vi "maincapactor1.vi"() -> ()   [LabVIEW 2024]
panel:
  out "dup directory path":path
  in  "GPIB address magnet":string
  in  "GPIB address Temp Controler":string
  in  "GPIB address CapBridge":string
  in  "Wait (minute)":u32
  in  "No of Temp Steps":i16
  in  "folder name to save files":string
  out "outputtemp":dbl[](array[numeric]) format="%.2f"
  out "outputdc":dbl[](array[numeric]) format="%.2f"
  out "outputcapacitor":dbl[](array[numeric]) format="%.2f"
  out "field":dbl[](array[numeric]) format="%.2f"
  out "Current Temp":dbl format="%.3f"
  in  "Increasing \nTemp step":bool=TRUE
  in  "Temperature\nInterval":dbl format="%.3f"
  in  "Initial Temp C":dbl format="%.3f"
  # "Help:\n1. write the folder name to save the files.The file name will \nbe the temperature in the given folder.\n2.Write the GPIB address of all the instruments before running\nthe program.\n3. Give the initial temperature and the temperature interval \nand the total number of steps.\n4.Check whether you want to increase the temperature or\ndecrease.\n5.Write the time to be waited to let the tempetature controller\nequilibrate.\n6.Once the speps 1 through 5 is done run the experiment."
  # "Decreasing\nTemp Step"
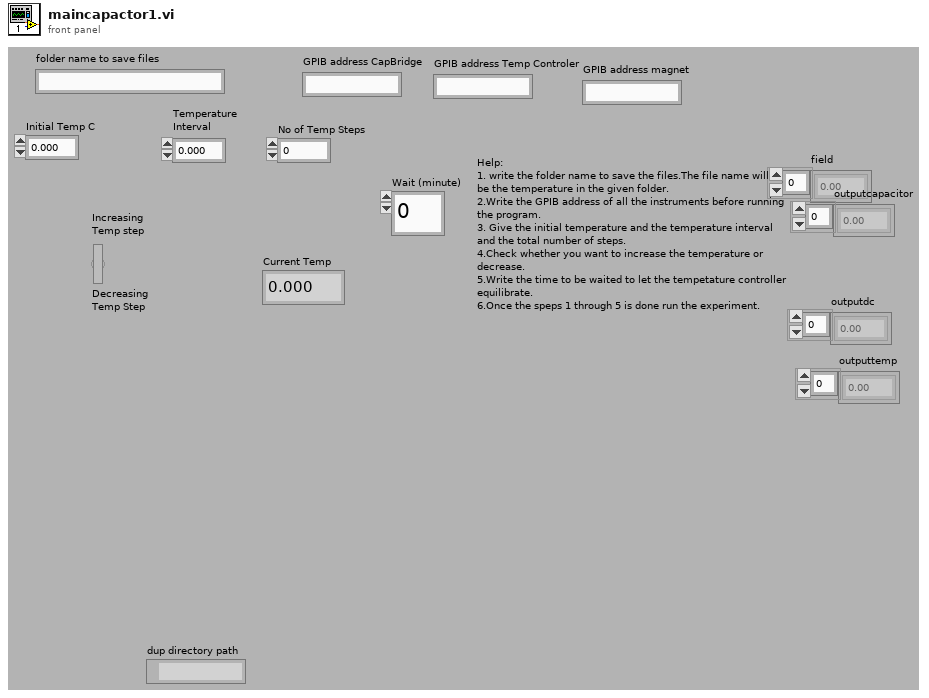
[diagram p1: front panel]
types:
  T1 = enum16{"--Quit--", "Read-Status", "Read-Cell", "Read-Field[T]", "Read-Setpoint[T]"}
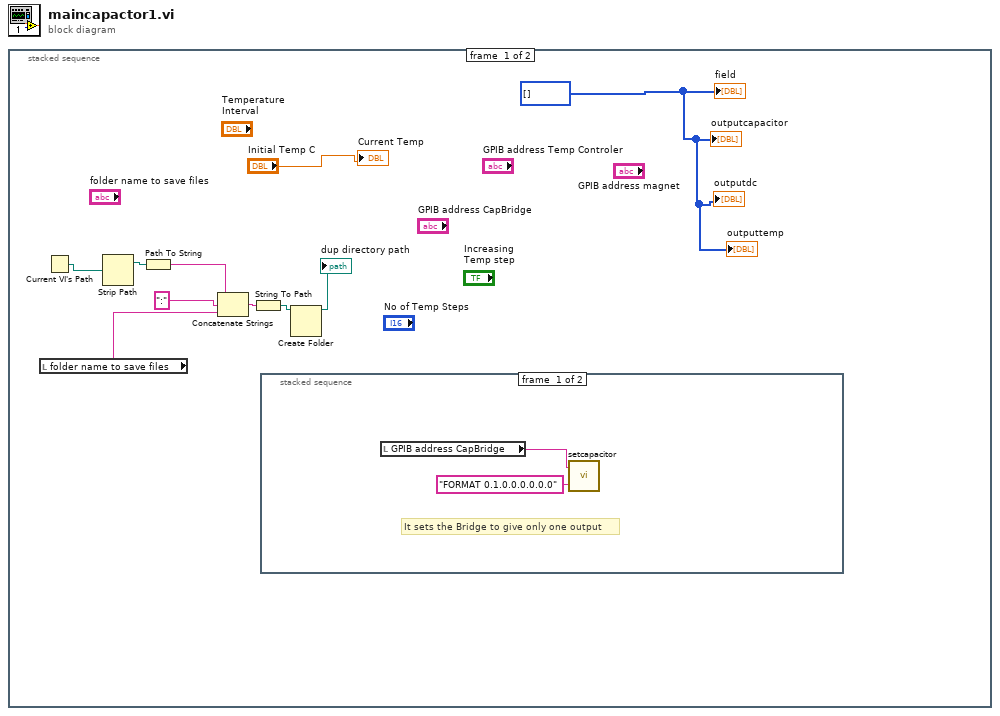
[diagram p0: block diagram]
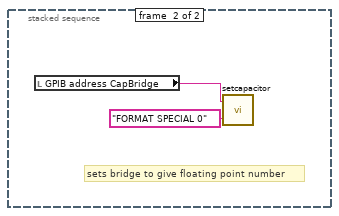
[diagram p2: hidden frame]
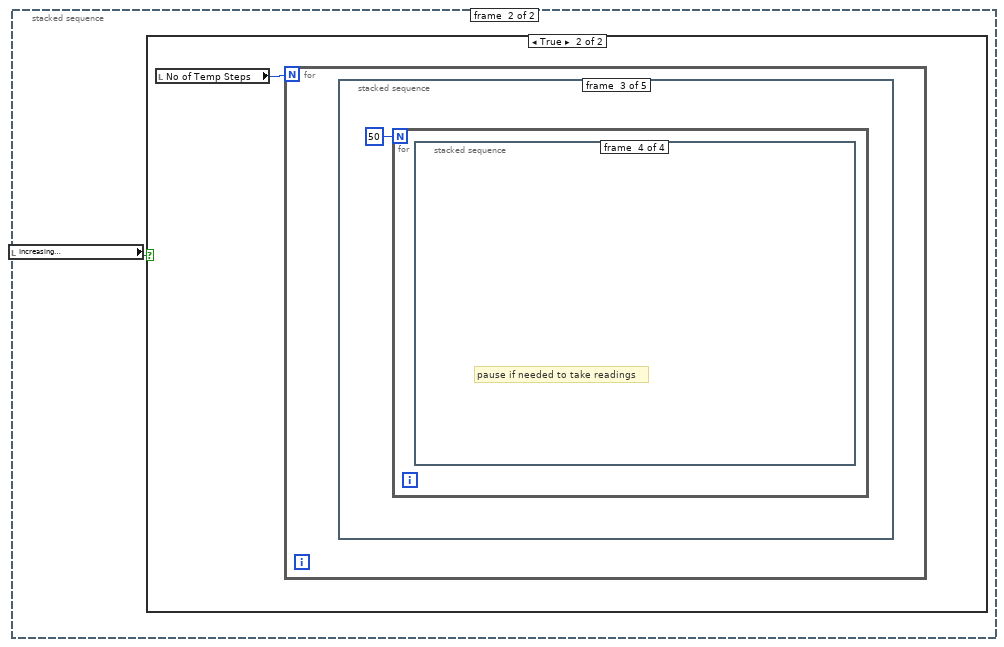
[diagram p3: hidden frame]
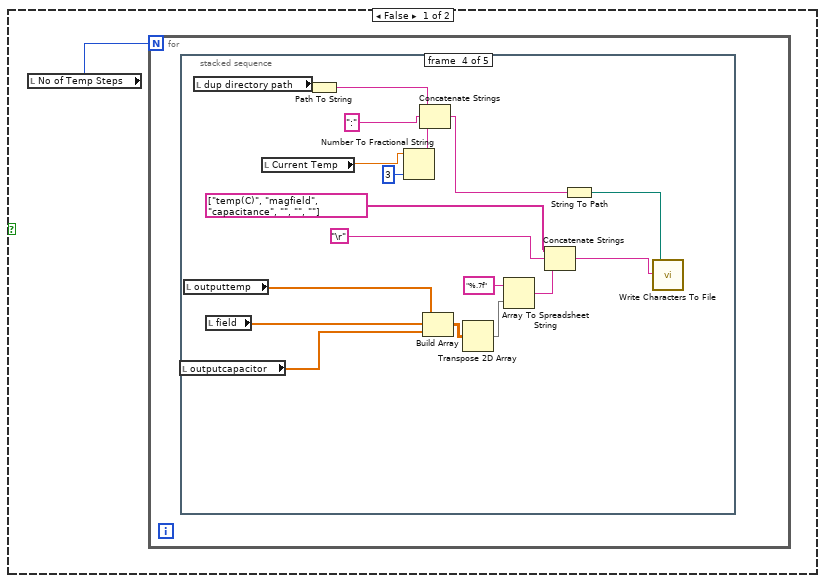
[diagram p4: hidden frame]
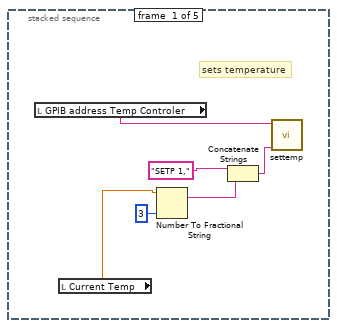
[diagram p5: hidden frame]
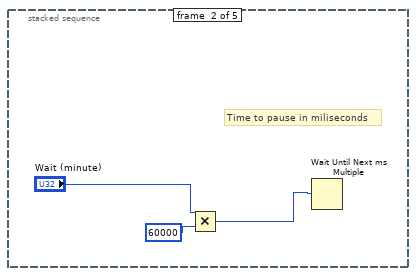
[diagram p6: hidden frame]
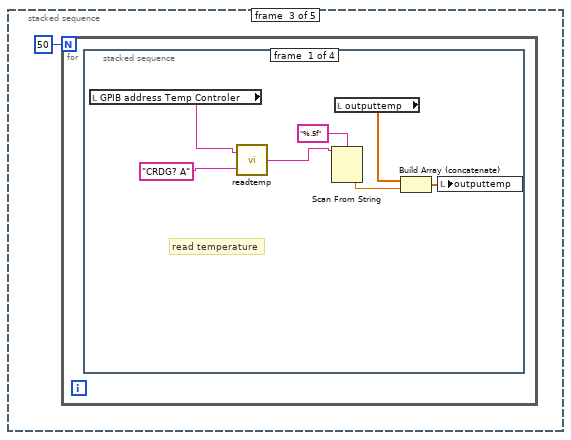
[diagram p7: hidden frame]
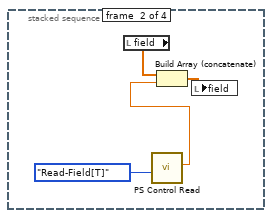
[diagram p8: hidden frame]
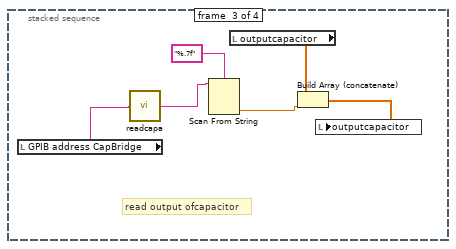
[diagram p9: hidden frame]
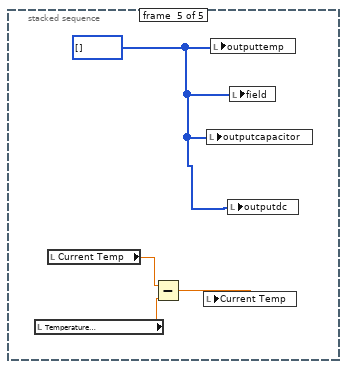
[diagram p11: hidden frame]
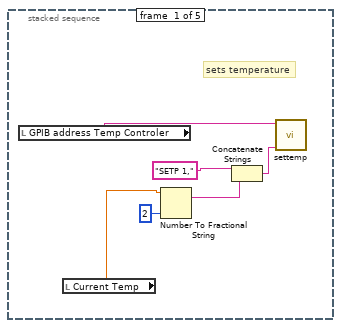
[diagram p12: hidden frame]
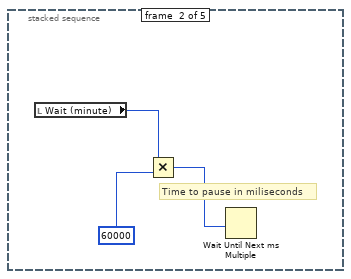
[diagram p13: hidden frame]
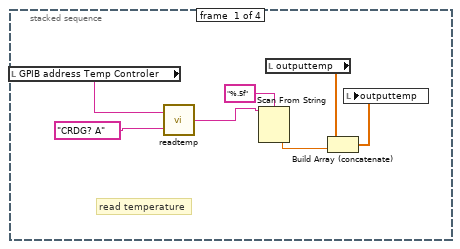
[diagram p14: hidden frame]
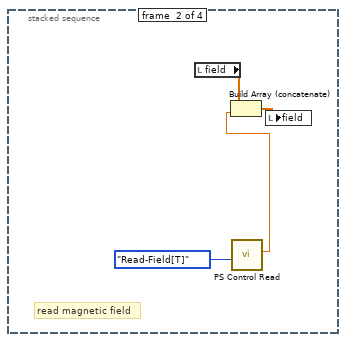
[diagram p15: hidden frame]
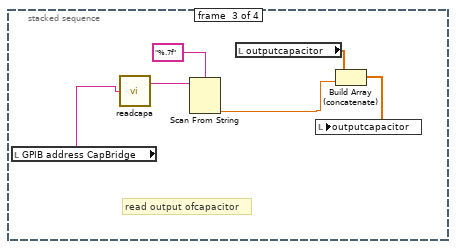
[diagram p16: hidden frame]
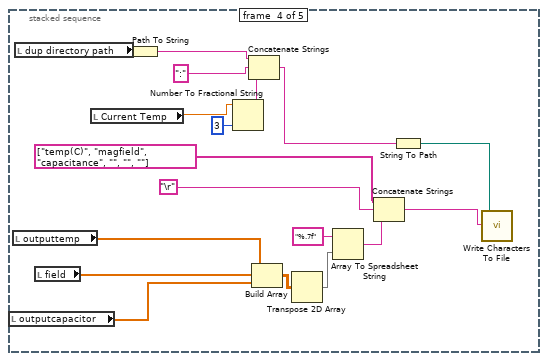
[diagram p17: hidden frame]
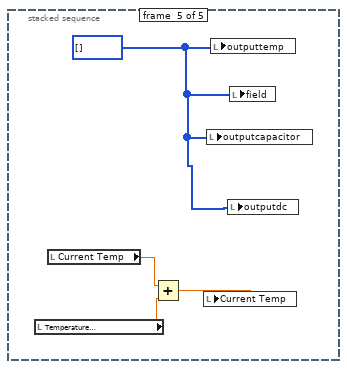
[diagram p18: hidden frame]
diagram:
  n1 = stacked-sequence {
    frame #0 {
      w9 = i32[] [] ("field")
      n2 = local read "folder name to save files"() -> (w4:string)
      n3 = Current VI's Path() -> (path=w8:path)
      n4 = Strip Path(path=w8) -> (stripped path=w7:path)  [unwired: 1 out]
      n5 = Path To String(path=w7) -> (string=w6:string)
      n6 = Concatenate Strings(w6, ":", w4) -> (w3:string)
      n7 = String To Path(string=w3) -> (path=w2:path)
      n8 = stacked-sequence {
        frame #0 {
          # "It sets the Bridge to give only one output"
          n9 = local read "GPIB address CapBridge"() -> (w12:string)
          n10 = call "setcapacitor.vi"("Characters to Write"="FORMAT 0.1.0.0.0.0.0.0", "GPIB\nAddress"=w12) -> ()  [unwired: 1 out]
        }
        frame #1 {
          # "sets bridge to give floating point number"
          n11 = local read "GPIB address CapBridge"() -> (w14:string)
          n12 = call "setcapacitor.vi"("Characters to Write"="FORMAT SPECIAL 0", "GPIB\nAddress"=w14) -> ()  [unwired: 1 out]
        }
      }
      n13 = Create Folder(path (use dialog)=w2) -> (created path=→"dup directory path":path)  [unwired: 2 in, 2 out]
      "Current Temp" <- "Initial Temp C"
      "field" <- w9
      "outputcapacitor" <- w9
      "outputdc" <- w9
      "outputtemp" <- w9
    }
    frame #1 {
      n14 = local read "Increasing \nTemp step"() -> (w15:bool)
      n15 = case shown="True" w15 {
        frame False {
          n16 = local read "No of Temp Steps"() -> (w16:i16)
          n17 = for {
            N: w16 -> [_]
            n18 = stacked-sequence {
              frame #0 {
                # "sets temperature"
                n19 = local read "GPIB address Temp Controler"() -> (w17:string)
                n20 = local read "Current Temp"() -> (w19:dbl)
                n21 = Number To Fractional String(number=w19, precision (6)=i16 3) -> (F-format string=w22:string)  [unwired: 2 in]
                n22 = Concatenate Strings("SETP 1,", w22) -> (w20:string)
                n23 = call "settemp.vi"("Characters to Write"=w20, "GPIB\nAddress"=w17) -> ()  [unwired: 5 in, 1 out]
              }
              frame #1 {
                # "Time to pause in miliseconds"
                n24 = Multiply(x="Wait (minute)", y=60000) -> (x*y=w23:u32)
                n25 = Wait Until Next ms Multiple(millisecond multiple=w23) -> ()  [unwired: 1 out]
              }
              frame #2 {
                n26 = for {
                  N: 50 -> [_]
                  n27 = stacked-sequence {
                    frame #0 {
                      # "read temperature"
                      n28 = local read "GPIB address Temp Controler"() -> (w29:string)
                      n29 = call "readtemp.vi"("Characters to Write"="CRDG? A", "GPIB\nAddress"=w29) -> ("Characters Read"=w30:string)
                      n30 = Scan From String(format string="%.5f", input string=w30) -> (output 1=w27:dbl)  [unwired: 3 in, 3 out]
                      n31 = local read "outputtemp"() -> (w28:dbl[])
                      n32 = Build Array (concatenate)(w28, w27) -> (w33:dbl[])
                      n33 = local write "outputtemp"(w33) -> ()
                    }
                    frame #1 {
                      n34 = local read "field"() -> (w36:dbl[])
                      n35 = call "PS Control Read.vi"("Read State"=T1."Read-Field[T]") -> ("Current Field"=w34:dbl)  [unwired: 3 in, 4 out]
                      n36 = Build Array (concatenate)(w36, w34) -> (w37:dbl[])
                      n37 = local write "field"(w37) -> ()
                    }
                    frame #2 {
                      # "read output ofcapacitor"
                      n38 = local read "GPIB address CapBridge"() -> (w40:string)
                      n39 = call "readcapa.vi"("GPIB\nAddress"=w40) -> ("Characters Read"=w41:string)
                      n40 = Scan From String(format string="%.7f", input string=w41) -> (output 1=w38:dbl)  [unwired: 3 in, 3 out]
                      n41 = local read "outputcapacitor"() -> (w39:dbl[])
                      n42 = Build Array (concatenate)(w39, w38) -> (w43:dbl[])
                      n43 = local write "outputcapacitor"(w43) -> ()
                    }
                    frame #3 {
                      # "pause if needed"
                    }
                  }
                }
              }
              frame #3 {
                n44 = local read "outputcapacitor"() -> (w46:dbl[])
                n45 = local read "outputtemp"() -> (w56:dbl[])
                n46 = local read "dup directory path"() -> (w45:path)
                n47 = local read "field"() -> (w55:dbl[])
                n48 = local read "Current Temp"() -> (w58:dbl)
                n49 = Path To String(path=w45) -> (string=w44:string)
                n50 = Number To Fractional String(number=w58, precision (6)=i16 3) -> (F-format string=w57:string)  [unwired: 2 in]
                n51 = Concatenate Strings(w44, ":", w57) -> (w60:string)
                n52 = Build Array(w56, w55, w46) -> (w54:dbl[][])
                n53 = Transpose 2D Array(2D array=w54) -> (transposed array=w52:dbl[][])
                n54 = Array To Spreadsheet String(array=w52, 3:"%.7f" ("format string")) -> (spreadsheet string=w49:string)  [unwired: 1 in]
                n55 = Concatenate Strings(string[] ["temp(C)", "magfield", "capacitance", "", "", ""], "\r", w49) -> (w48:string)
                n56 = String To Path(string=w60) -> (path=w59:path)
                n57 = call <vilib>:"Write Characters To File.vi"("character string"=w48, "file path (dialog if empty)"=w59) -> ()  [unwired: 3 in, 1 out]
              }
              frame #4 {
                w65 = i32[] []
                n58 = local read "Temperature\nInterval"() -> (w63:dbl)
                n59 = local read "Current Temp"() -> (w64:dbl)
                n60 = Subtract(x=w64, y=w63) -> (x-y=w62:dbl)
                n61 = local write "Current Temp"(w62) -> ()
                n62 = local write "outputcapacitor"(w65) -> ()
                n63 = local write "outputtemp"(w65) -> ()
                n64 = local write "outputdc"(w65) -> ()
                n65 = local write "field"(w65) -> ()
              }
            }
          }
        }
        frame True {
          n66 = local read "No of Temp Steps"() -> (w66:i16)
          n67 = for {
            N: w66 -> [_]
            n68 = stacked-sequence {
              frame #0 {
                # "sets temperature"
                n69 = local read "GPIB address Temp Controler"() -> (w67:string)
                n70 = local read "Current Temp"() -> (w69:dbl)
                n71 = Number To Fractional String(number=w69, precision (6)=i16 2) -> (F-format string=w72:string)  [unwired: 2 in]
                n72 = Concatenate Strings("SETP 1,", w72) -> (w70:string)
                n73 = call "settemp.vi"("Characters to Write"=w70, "GPIB\nAddress"=w67) -> ()  [unwired: 5 in, 1 out]
              }
              frame #1 {
                # "Time to pause in miliseconds"
                n74 = local read "Wait (minute)"() -> (w75:u32)
                n75 = Multiply(x=w75, y=u32 60000 ("millisecond multiple")) -> (x*y=w73:u32)
                n76 = Wait Until Next ms Multiple(millisecond multiple=w73) -> ()  [unwired: 1 out]
              }
              frame #2 {
                n77 = for {
                  N: 50 -> [_]
                  n78 = stacked-sequence {
                    frame #0 {
                      # "read temperature"
                      n79 = local read "GPIB address Temp Controler"() -> (w79:string)
                      n80 = call "readtemp.vi"("Characters to Write"="CRDG? A", "GPIB\nAddress"=w79) -> ("Characters Read"=w80:string)
                      n81 = Scan From String(format string="%.5f", input string=w80) -> (output 1=w77:dbl)  [unwired: 3 in, 3 out]
                      n82 = local read "outputtemp"() -> (w78:dbl[])
                      n83 = Build Array (concatenate)(w78, w77) -> (w83:dbl[])
                      n84 = local write "outputtemp"(w83) -> ()
                    }
                    frame #1 {
                      # "read magnetic field"
                      n85 = local read "field"() -> (w86:dbl[])
                      n86 = call "PS Control Read.vi"("Read State"=T1."Read-Field[T]") -> ("Current Field"=w84:dbl)  [unwired: 3 in, 4 out]
                      n87 = Build Array (concatenate)(w86, w84) -> (w87:dbl[])
                      n88 = local write "field"(w87) -> ()
                    }
                    frame #2 {
                      # "read output ofcapacitor"
                      n89 = local read "GPIB address CapBridge"() -> (w90:string)
                      n90 = call "readcapa.vi"("GPIB\nAddress"=w90) -> ("Characters Read"=w91:string)
                      n91 = Scan From String(format string="%.7f", input string=w91) -> (output 1=w88:dbl)  [unwired: 3 in, 3 out]
                      n92 = local read "outputcapacitor"() -> (w89:dbl[])
                      n93 = Build Array (concatenate)(w89, w88) -> (w93:dbl[])
                      n94 = local write "outputcapacitor"(w93) -> ()
                    }
                    frame #3 {
                      # "pause if needed to take readings"
                    }
                  }
                }
              }
              frame #3 {
                n95 = local read "outputcapacitor"() -> (w96:dbl[])
                n96 = local read "outputtemp"() -> (w106:dbl[])
                n97 = local read "dup directory path"() -> (w95:path)
                n98 = local read "field"() -> (w105:dbl[])
                n99 = local read "Current Temp"() -> (w108:dbl)
                n100 = Path To String(path=w95) -> (string=w94:string)
                n101 = Number To Fractional String(number=w108, precision (6)=i16 3) -> (F-format string=w107:string)  [unwired: 2 in]
                n102 = Concatenate Strings(w94, ":", w107) -> (w110:string)
                n103 = Build Array(w106, w105, w96) -> (w104:dbl[][])
                n104 = Transpose 2D Array(2D array=w104) -> (transposed array=w102:dbl[][])
                n105 = Array To Spreadsheet String(array=w102, 3:"%.7f" ("format string")) -> (spreadsheet string=w99:string)  [unwired: 1 in]
                n106 = Concatenate Strings(string[] ["temp(C)", "magfield", "capacitance", "", "", ""], "\r", w99) -> (w98:string)
                n107 = String To Path(string=w110) -> (path=w109:path)
                n108 = call <vilib>:"Write Characters To File.vi"("character string"=w98, "file path (dialog if empty)"=w109) -> ()  [unwired: 3 in, 1 out]
              }
              frame #4 {
                w115 = i32[] []
                n109 = local read "Temperature\nInterval"() -> (w113:dbl)
                n110 = local read "Current Temp"() -> (w114:dbl)
                n111 = Add(x=w114, y=w113) -> (x+y=w112:dbl)
                n112 = local write "Current Temp"(w112) -> ()
                n113 = local write "outputcapacitor"(w115) -> ()
                n114 = local write "outputtemp"(w115) -> ()
                n115 = local write "outputdc"(w115) -> ()
                n116 = local write "field"(w115) -> ()
              }
            }
          }
        }
      }
    }
  }
